vi "reset-class-data.vi"(8 "error in (no error)":errorcluster, 11 "CANtable in":refnum<class "dbc.lvclass">) -> (0 "error out":errorcluster, 3 "CANtable out":refnum<class "dbc.lvclass">)   [LabVIEW 2015, in "dbc.lvclass"]
uses:
  dbc.lvclass
  dbc.lvclass/dbc.ctl
  controls/dbc-content-data.ctl
  controls/dbc-active-item.ctl
  class.bFrameIO/bFrameIO.lvclass
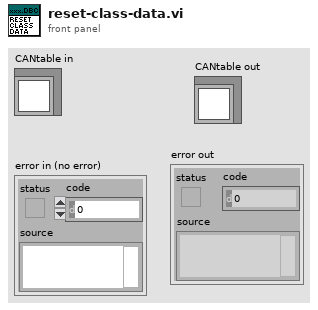
[diagram p1: front panel]
types:
  T1 = typedef "dbc-active-item.ctl" = cluster{"active.frame.tag":string, "activeItemTag":string, "indent.lvl":i32, "symbol":i32}
  T2 = typedef "dbc-content-data.ctl" = cluster{"Number of Clusters":i32, "Number of Frames ":i32[], "Clusters":string[], "Frames":string[][], "Signals":string[][][], "Number of Signals":i32[][]}
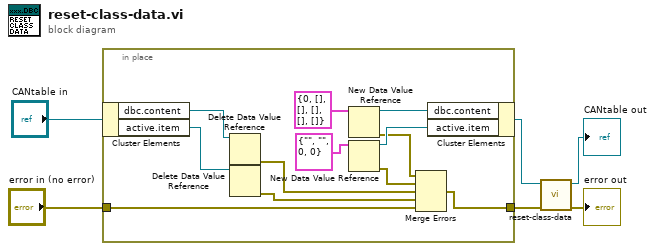
[diagram p0: block diagram]
diagram:
  n1 = in-place {
    in-place-border: [w16] -> w2
    in-place-border: "error in (no error)" -> [w15]
    n2 = in-place-cluster #1("CANtable in") -> ("dbc.content"=w14:refnum<data-value>, "active.item"=w17:refnum<data-value>)
    n3 = Delete Data Value Reference(data value reference=w14) -> (error out=w13:errorcluster)  [unwired: 1 in, 1 out]
    n4 = Delete Data Value Reference(data value reference=w17) -> (error out=w18:errorcluster)  [unwired: 1 in, 1 out]
    n5 = New Data Value Reference(data value=T2 {"Number of Clusters"=0, "Number of Frames "=[], "Clusters"=[], "Frames"=[], "Signals"=[], "Number of Signals"=[]} ("Cluster")) -> (data value reference=w10:refnum<data-value>, error out=w7:errorcluster)  [unwired: 1 in]
    n6 = New Data Value Reference(data value=T1 {"active.frame.tag"="", "activeItemTag"="", "indent.lvl"=0, "symbol"=0} ("active.item")) -> (data value reference=w9:refnum<data-value>, error out=w8:errorcluster)  [unwired: 1 in]
    n7 = Merge Errors(w7, w8, w13, w18, w15) -> (w16:errorcluster)
    n8 = in-place-cluster #1("dbc.content"=w10, "active.item"=w9) -> (w3:refnum<class "dbc.lvclass">)
  }
  n9 = call-parent "reset-class-data.vi"("error in (no error)"=w2, "CANtable in"=w3) -> ("error out"=→"error out":errorcluster, "CANtable out"=→"CANtable out":refnum<class "dbc.lvclass">)  [unwired: 8 in]
